vi "test-scene-window.vi"() -> ()   [LabVIEW 2013]
uses:
  <vilib>/Utility/miscctls.llb/LVRectTypeDef.ctl
  <vilib>/picture/3D Picture Control/NI_3D Picture Control.lvlib
panel:
  in  "停止按钮":bool
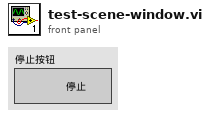
[diagram p1: front panel]
types:
  T1 = enum16{"Open", "Minimized", "Maximized", "Hidden"}
  T2 = typedef "LVRectTypeDef.ctl" = cluster{"Left":i16, "Top":i16, "Right":i16, "Bottom":i16}
  T3 = enum16{"None", "Spherical", "Flying", "Oriented"}
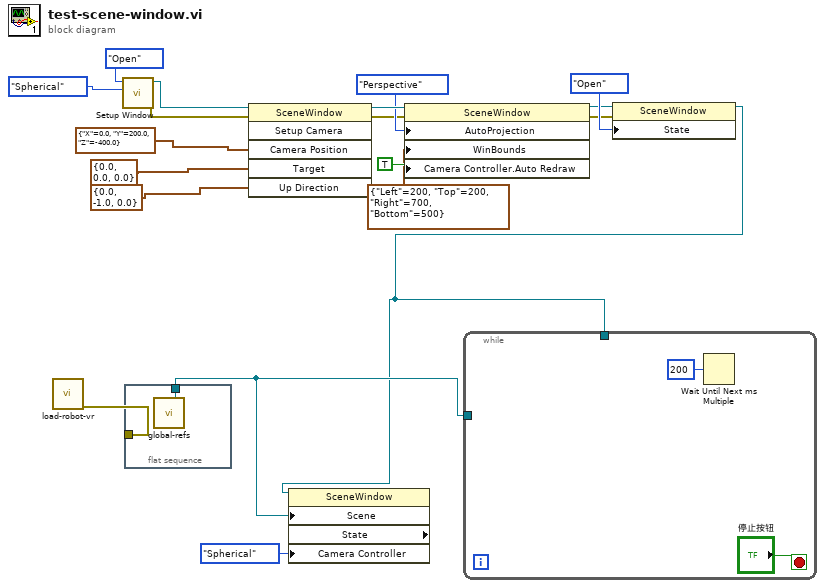
[diagram p0: block diagram]
diagram:
  n1 = call "load-robot-vr.vi"() -> ("错误输出"=w17:errorcluster)  [unwired: 11 in]
  n2 = call <vilib>:"Setup Window.vi"("Camera Controller"=enum16{"None", "Spherical", "Flying"}."Spherical", "Window State"=T1."Open") -> ("error out"=w2:errorcluster, "New Window Refnum"=w3:refnum<vi>)  [unwired: 1 in, 7 out]
  n3 = flat-sequence {
    tunnel: [w20] -> w15
    tunnel: w17 -> [_]
    frame #0 {
      n4 = call "global-refs.vi"() -> ("RobotRef"=w20:refnum<vi>)  [unwired: 10 in, 5 out]
    }
  }
  n5 = invoke class="SceneWindow" method="Setup Camera"(reference=w3, error in=w2, "Camera Position"=cluster{"X":sgl, "Y":sgl, "Z":sgl} {"X"=0.0, "Y"=200.0, "Z"=-400.0}, "Target"=cluster{"X":sgl, "Y":sgl, "Z":sgl} {"X"=0.0, "Y"=0.0, "Z"=0.0}, "Up Direction"=cluster{"X":sgl, "Y":sgl, "Z":sgl} {"X"=0.0, "Y"=-1.0, "Z"=0.0}) -> (reference out=w12:refnum<vi>, error out=w8:errorcluster)  [unwired: 1 in, 4 out]
  n6 = property class="SceneWindow"(reference=w12, error in=w8, "AutoProjection"=enum16{"None", "Perspective", "Orthographic"}."Perspective" ("Automatic Projection Mode"), "WinBounds"=T2 {"Left"=200, "Top"=200, "Right"=700, "Bottom"=500} ("Window Bounds"), "Camera Controller.Auto Redraw"=TRUE ("Camera Controller:Auto Redraw")) -> (reference out=w9:refnum<vi>, error out=w7:errorcluster)
  n7 = property class="SceneWindow"(reference=w9, error in=w7, "State"=T1."Open" ("Window State")) -> (reference out=w1:refnum<vi>)  [unwired: 1 out]
  n8 = property class="SceneWindow" props=["Scene", "State", "Camera Controller"](reference=w1, "Scene"=w15, "Camera Controller"=T3."Spherical" ("视角控制器:类型")) -> ()  [unwired: 1 in, 3 out]
  n9 = while {
    tunnel: w1 -> [_]
    tunnel: w15 -> [_]
    stop <- "停止按钮" stop-if-true
    n10 = Wait Until Next ms Multiple(millisecond multiple=u32 200 ("毫秒倍数")) -> ()  [unwired: 1 out]
  }
